vi "Output BPM.vi"(4 "error in (no error)":errorcluster, 7 "BPM (input)":dbl) -> (0 "error out":errorcluster, 3 "BPM (output)":string)   [LabVIEW 2020]
doc: "Takes the BPM input and outputs the BPM as a string after a certain number of samples, otherwise the VI returns the \"Calibrating...\" message as the filter may still be settling"
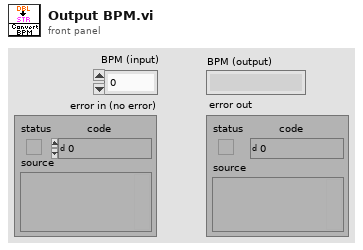
[diagram p1: front panel]
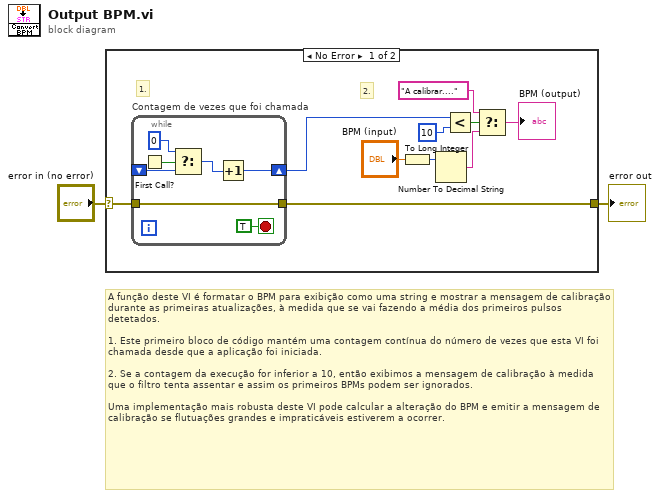
[diagram p0: block diagram]
diagram:
  # "A função deste VI é formatar o BPM para exibição como uma string e mostrar a mensagem de calibração durante as primeiras atualizações, à medida que se vai fazendo a média dos primeiros pulsos detetados.\n\n1. Este primeiro bloco de código mantém uma contagem contínua do número de vezes que esta VI foi chamada desde que a aplicação foi iniciada. \n\n2. Se a contagem da execução for inferior a 10, então exibimos a mensagem de calibração à medida que o filtro tenta assentar e assim os primeiros BPMs podem ser ignorados.\n\nUma implementação mais robusta deste VI pode calcular a alteração do BPM e emitir a mensagem de calibração se flutuações grandes e impraticáveis estiverem a ocorrer."
  n1 = case shown="No Error" "error in (no error)" {
    selector: "error in (no error)" -> [w3 w20]
    tunnel: [w12 w20] -> w2
    frame No Error {
      # "2."
      # "1."
      n2 = while "Contagem de vezes que foi chamada" {
        shift-right: [w18] -> w4
        shift-left: _ -> [w14]
        tunnel: w3 -> [w17]
        tunnel: [w17] -> w12
        stop <- TRUE stop-if-true
        n3 = First Call?() -> (First Call?: T/F=w16:bool)
        n4 = Select(t=u64 0, s=w16, f=w14) -> (s? t:f=w13:u64)
        n5 = Increment(x=w13) -> (x+1=w18:u64)
      }
      n6 = To Long Integer(number="BPM (input)") -> (32bit integer=w9:i32)
      n7 = Number To Decimal String(number=w9) -> (decimal integer string=w6:string)  [unwired: 1 in]
      n8 = Less?(x=w4, y=u64 10) -> (x < y?=w11:bool)
      n9 = Select(t="A calibrar....", s=w11, f=w6) -> (s? t:f=→"BPM (output)":string)
    }
    frame Error {
    }
  }
  "error out" <- w2
